vi "ATSh_GetMaxPretriggerSamples.vi"(11 "HandleIn":u32) -> (0 "Return Code":u32, 1 "MaxPretriggerSamples":u32, 3 "HandleOut":u32)   [LabVIEW 2015]
doc: "_____AlazarTech, Scope_____\n\nGet the maximum Pretrigger Samples available."
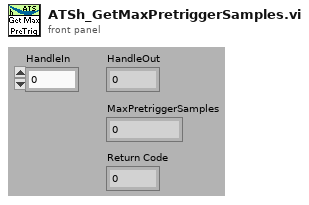
[diagram p1: front panel]
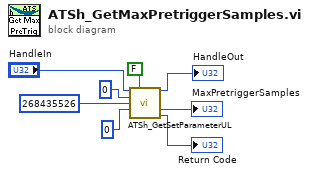
[diagram p0: block diagram]
diagram:
  n1 = call "ATSh_GetSetParameterUL.vi"("Handle"="HandleIn", "Get / Set&Get"=FALSE, "Channel"=u8 0, "Parameter"=u32 268435526, "Value"=u32 0) -> ("Handle_Out"=→"HandleOut":u32, "Value_Out"=→"MaxPretriggerSamples":u32, "Return Code"=→"Return Code":u32)  [unwired: 8 in]
